vi "DSF.Transceiver.UDP.Rx.vi"(8 "error in (no error)":errorcluster, 9 "Transfer Group Rx parameters":T1={"Transfers Rx"=[], "max size"=548} {"max size" format="%d bytes"; "Transfers Rx"."source address" format="%d ms"; "Transfers Rx"."timeout" format="%d bytes"}, 10 "Transfer Group":refnum<class "DSF.Engine.Transfer Group.lvclass">, 11 "UDP Transceiver in":refnum<class "DSF.Transceiver.UDP.lvclass">) -> (0 "error out":errorcluster, 3 "UDP Transceiver out":refnum<class "DSF.Transceiver.UDP.lvclass">)   [LabVIEW 2017, in "DSF.Transceiver.UDP.lvlib" / "DSF.Transceiver.UDP.lvclass"]
uses:
  DSF.Transceiver.UDP.lvclass
  DSF.Transceiver.UDP.Parameters.Transfer Group.Rx.ctl
  DSF.Transceiver.UDP.Parameters.Transfer.Rx.ctl
  DSF Core/Built/Engine/DSF.Engine.lvlibp/Engine/Classes/Transfer/DSF.Engine.Transfer Group.lvclass
  DSF.Transceiver.UDP.lvclass/DSF.Transceiver.UDP.ctl
  DSF.Transceiver.UDP.Errors.vi
  DSF.Transceiver.UDP.Errors.Rx.Unknown Datagram.vi
  DSF.Transceiver.UDP.Errors.Rx.Size Mismatch.vi
  <vilib>/NI/Static Error Handling/VIs/Static Error Handling.Source Buffer.Write.String.vi
  <vilib>/NI/Static Error Handling/VIs/Static Error Handling.Source Buffer.Write.Numeric.Scalar.Base10.vi
  <vilib>/NI/Static Error Handling/VIs/Static Error Handling.Source Buffer.Write.Numeric.Scalar.Base10 (U16).vi
  <vilib>/NI/Static Error Handling/VIs/Static Error Handling.Source Buffer.Write.Numeric.Scalar.Base10 (U64).vi
  DSF Core/Built/Engine/DSF.Engine.lvlibp/Engine/Classes/Buffer/DSF.Engine.Memory.Buffer.Write.vi
  DSF Core/Built/Engine/DSF.Engine.lvlibp/Engine/Classes/Buffer/DSF.Engine.Memory.Buffer.Write.1D.U8.vi
  DSF.Transceiver.UDP.Error.Create.vi
  DSF Core/Built/Engine/DSF.Engine.lvlibp/Engine/Classes/Buffer/DSF.Engine.Memory.Buffer.Get Buffer Size.vi
  DSF Core/Built/Engine/DSF.Engine.lvlibp/Engine/Classes/Transfer/DSF.Engine.Transfer.Get String Buffer.vi
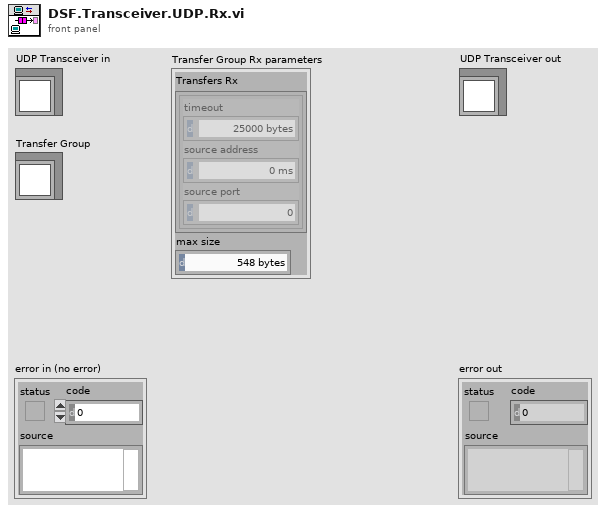
[diagram p1: front panel]
types:
  T1 = typedef "DSF.Transceiver.UDP.lvlib/DSF.Transceiver.UDP.lvclass/DSF.Transceiver.UDP.Parameters.Transfer Group.Rx.ctl" = cluster{"Transfers Rx":T2[], "max size":i32}
  T2 = typedef "DSF.Transceiver.UDP.lvlib/DSF.Transceiver.UDP.lvclass/DSF.Transceiver.UDP.Parameters.Transfer.Rx.ctl" = cluster{"timeout":i32, "source address":u32, "source port":u16}
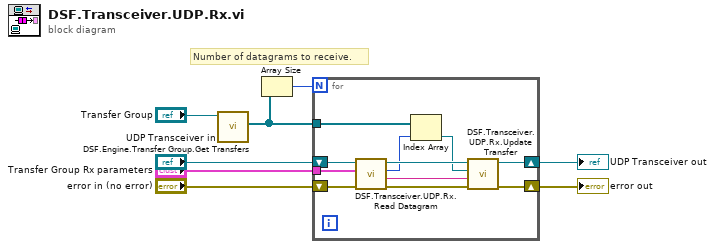
[diagram p0: block diagram]
diagram:
  # "Number of datagrams to receive."
  n1 = call "DSF.Engine.Transfer Group.Get Transfers.vi"("Transfer Group in"="Transfer Group") -> ("Transfers"=w3:refnum<class "DSF.Engine.Transfer.lvclass">[])  [unwired: 9 in, 1 out]
  n2 = Array Size(array=w3) -> (size(s)=w4:i32)
  n3 = for {
    N: w4 -> [_]
    shift-right: [w9] -> w6
    shift-left: "error in (no error)" -> [w18]
    tunnel: w3 -> [w16]
    tunnel: "Transfer Group Rx parameters" -> [w17]
    shift-right: [w10] -> w1
    shift-left: "UDP Transceiver in" -> [w19]
    n4 = call "DSF.Transceiver.UDP.Rx.Read Datagram.vi"("error in (no error)"=w18, "Transfer Group Rx parameters"=w17, "UDP Transceiver in"=w19) -> ("error out"=w14:errorcluster, "data"=w13:string, "Transfer index"=w11:i32, "UDP Transceiver out"=w15:refnum<class "DSF.Transceiver.UDP.lvclass">)  [unwired: 5 in]
    n5 = Index Array(array=w16, index=w11) -> (element=w12:refnum<class "DSF.Engine.Transfer.lvclass">)
    n6 = call "DSF.Transceiver.UDP.Rx.Update Transfer.vi"("error in (no error)"=w14, "data"=w13, "Transfer"=w12, "UDP Transceiver in"=w15) -> ("error out"=w9:errorcluster, "UDP Transceiver out"=w10:refnum<class "DSF.Transceiver.UDP.lvclass">)  [unwired: 6 in]
  }
  "error out" <- w6
  "UDP Transceiver out" <- w1
